vi "5-Axis (Manual).vi"() -> ()   [LabVIEW 2014]
uses:
  EMC API/EMC_Typedef_Motor_Parameters.ctl
  Typedef/Typedef_Motor_Action.ctl
  Functional_Global/Typedef_FPGA_Interface_Action.ctl
  <vilib>/Motion/Express/_s/nimc.ex.clearFaults.clearFaults.axis.vi
  <vilib>/Motion/Express/_s/nimc.ex.power.power.axis.vi
  <vilib>/Motion/Express/_s/nimc.ex.resetPosition.resetPosition.axis.vi
  <vilib>/Utility/error.llb/Error Cluster From Error Code.vi
  <vilib>/rvi/errors/niLvFpgaAdjustHostInterfaceError.vi
  <vilib>/Motion/Express/_s/nimc.ex.read.readTrajectoryData.axis.vi
  <vilib>/Motion/Express/_s/nimc.ex.read.readMotionIO.axis.vi
  <vilib>/Motion/Express/_s/nimc.ex.findReferenceMove.startReferenceMove.axis.modeReverseLimit.vi
  <vilib>/Motion/Express/_s/nimc.ex.findReferenceMove.startReferenceMove.axis.modeHome.vi
  <vilib>/Motion/Express/_s/nimc.ex.findReferenceMove.startReferenceMove.axis.modeForwardLimit.vi
  <vilib>/Motion/BlockNode/FB.NIMotion.xnode
  <vilib>/rvi/interface/nirviReadWriteControl/nirviReadWriteControl.xnode
  NiFpgaLv.dll
  <vilib>/rvi/interface/Simulation/niFpgaSimulationCallBeginRW.vi
panel:
  out "Rev Limits":bool[](array[boolean])
  out "Fwd Limits":bool[](array[boolean])
  out "Home Limits":bool[](array[boolean])
  in  "Mod3/DIO28":bool
  in  "Mod3/DIO29":bool
  in  "Mod3/DIO30":bool
  in  "Mod3/DIO31":bool
  in  "resource":refnum<k21>="Axis 1"
  out "home active":bool
  out "rev. limit active":bool
  out "fwd. limit active":bool
  out "XY Graph":cluster{"X Array":dbl[], "Y Array":dbl[]}(graph)
  in  "interval":dbl=0.01 format="%#_13g"
  in  "Gear in/out":enum16{"Gear in", "Gear out"}(ring)
  in  "denominator":i32=1
  in  "numerator":i32=1
  in  "Master Axis":T1(ring)
  out "Array":dbl[](array[knob]) scale=0.0..1000.0
  in  "Clear Errors":bool
  in  "Command":T2
  in  "Motion Parameters":T3={"position"=1000.0, "velocity"=1000.0, "acceleration"=10000.0, "deceleration"=10000.0, "accel. jerk"=10000.0, "decel. jerk"=10000.0}
  in  "Axis Index":T1(ring)
  out "error":errorcluster
  out "Numeric":i32
  in  "Stop all motors":bool
  in  "Execute Command":bool
  in  "stop":bool
  out "Axis Velocities":T4(graph)
  out "Axis Positions":T4(graph)
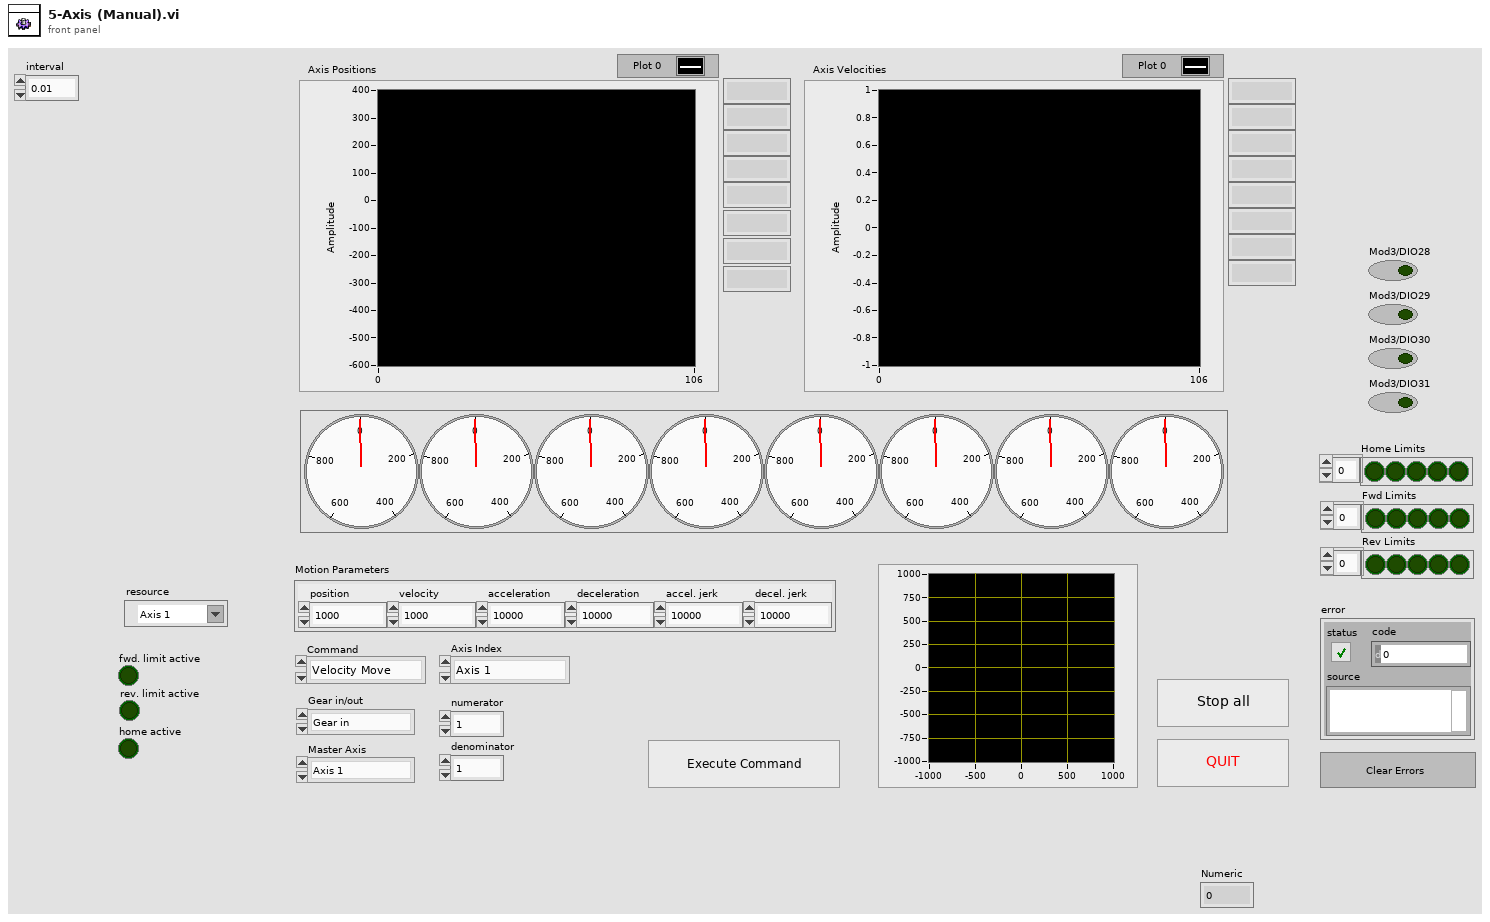
[diagram p1: front panel]
types:
  T1 = enum16{"Axis 1", "Axis 2", "Axis 3", "Axis 4", "Axis 5", "Axis 6", "Axis 7", "Axis 8"}
  T2 = typedef "Typedef_Motor_Action.ctl" = enum16{"Velocity Move", "REL Pos Move", "ABS Pos Move", "Stop", "Reset Position", "Coordinate_move", "Contour_move", "Gearing", "Find Fwd Limit", "Find Rev Limit", "Find Home"}
  T3 = typedef "EMC_Typedef_Motor_Parameters.ctl" = cluster{"position":dbl, "velocity":dbl, "acceleration":dbl, "deceleration":dbl, "accel. jerk":dbl, "decel. jerk":dbl}
  T4 = cluster{"[0]":dbl, "[1]":dbl, "[2]":dbl, "[3]":dbl, "[4]":dbl, "[5]":dbl, "[6]":dbl, "[7]":dbl}
  T5 = typedef "Typedef_FPGA_Interface_Action.ctl" = enum16{"Initialize FPGA", "Get FPGA Reference", "Close FPGA"}
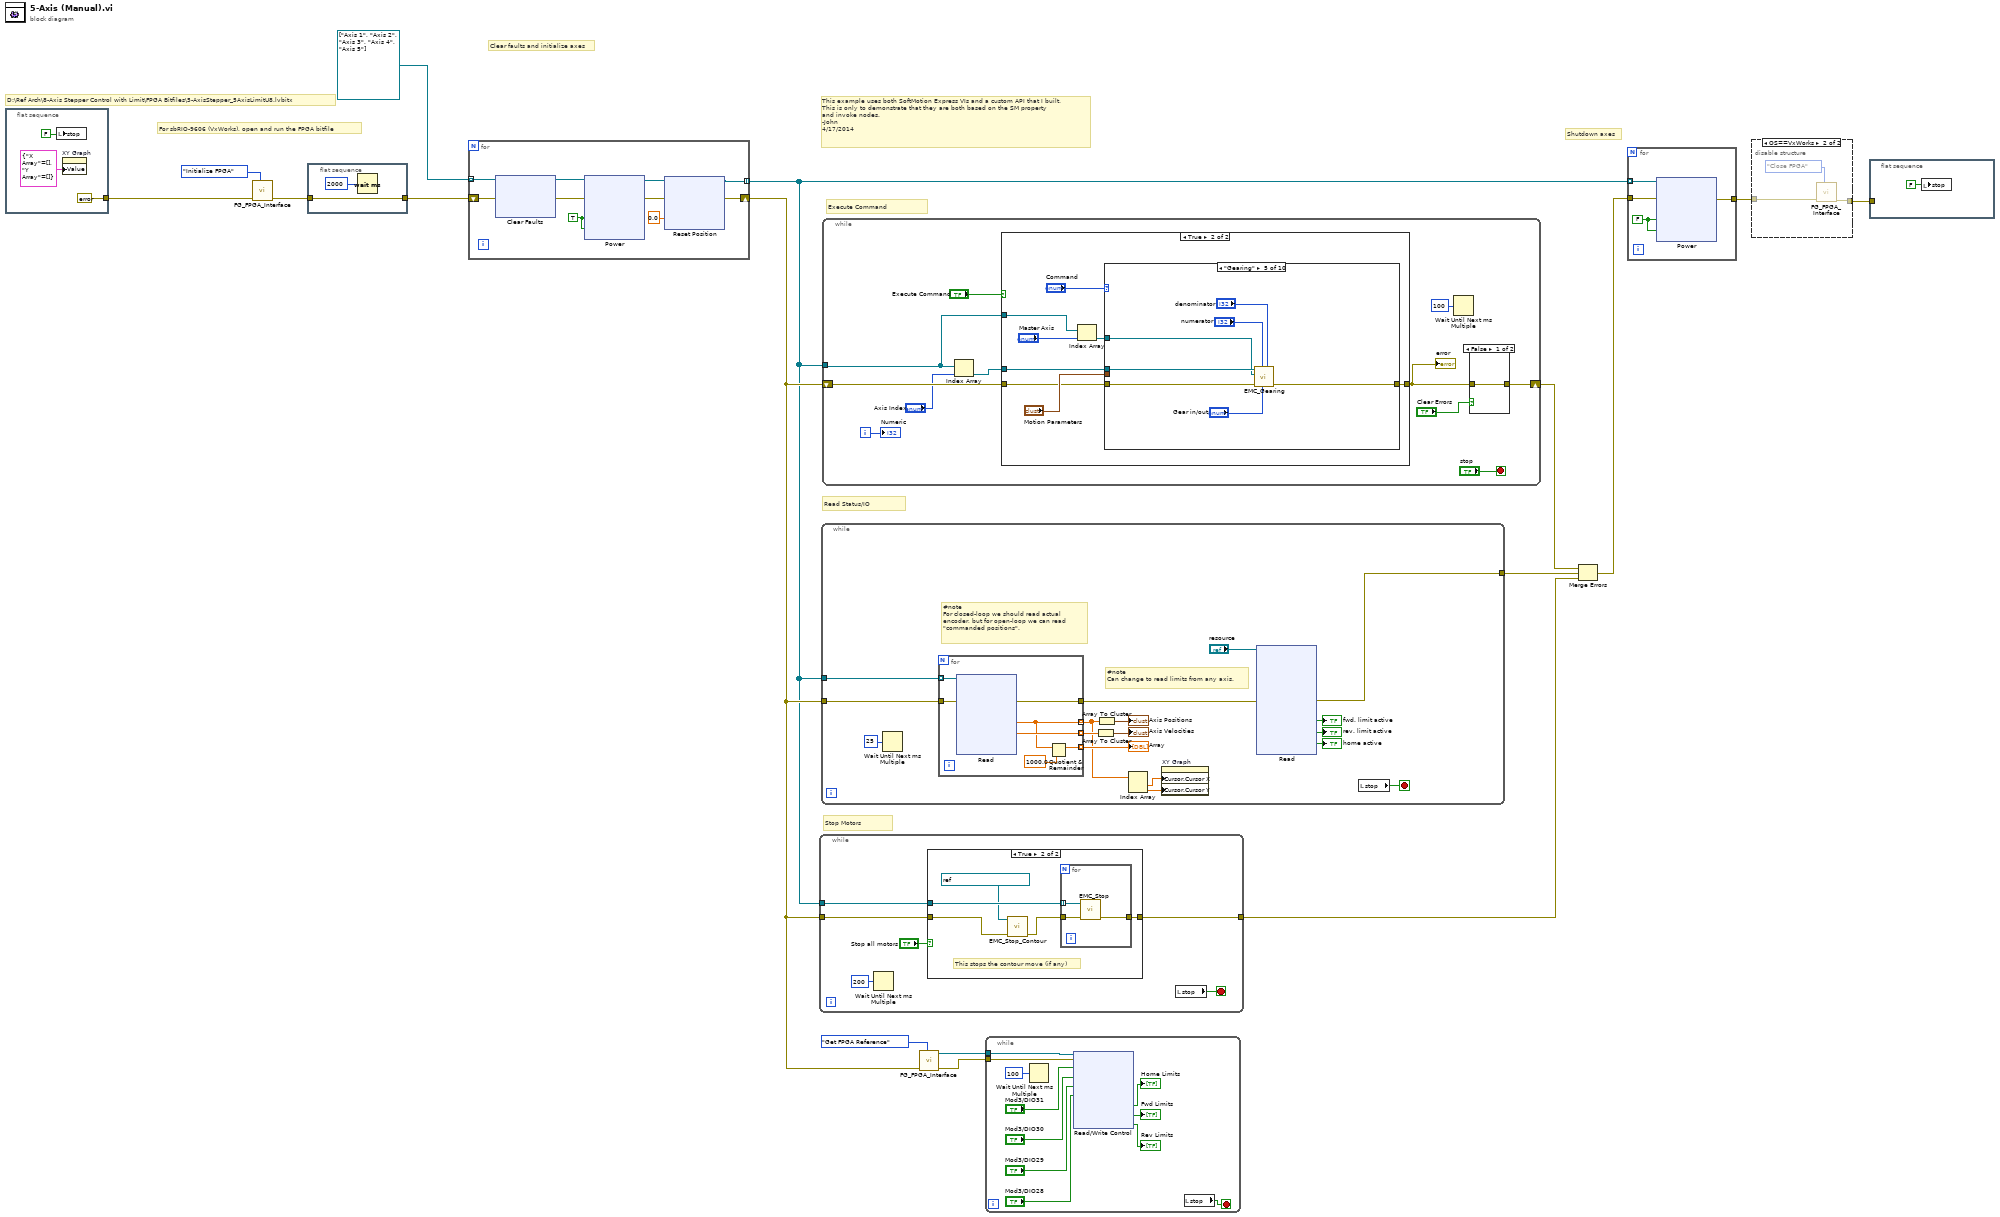
[diagram p0: block diagram]
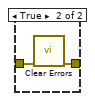
[diagram p4: hidden frame]
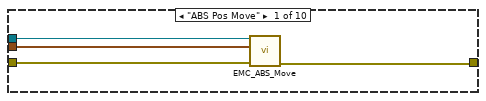
[diagram p6: hidden frame]
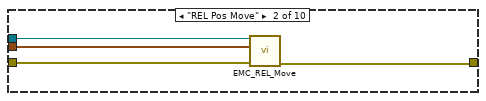
[diagram p7: hidden frame]
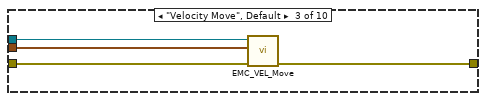
[diagram p8: hidden frame]
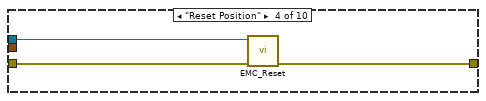
[diagram p9: hidden frame]
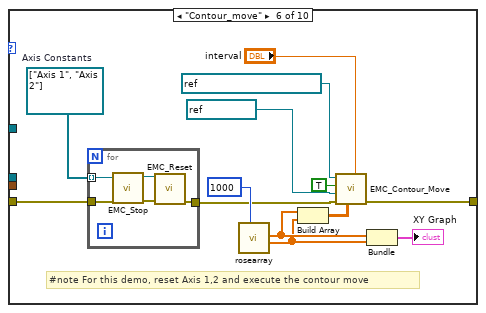
[diagram p10: hidden frame]
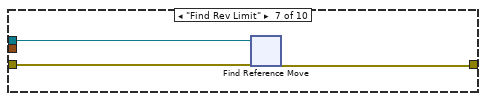
[diagram p11: hidden frame]
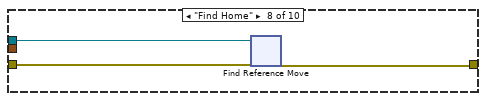
[diagram p12: hidden frame]
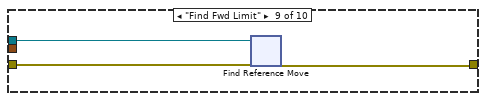
[diagram p13: hidden frame]
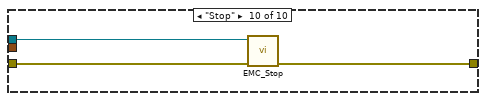
[diagram p14: hidden frame]
diagram:
  # "For sbRIO-9606 (VxWorks), open and run the FPGA bitfile"
  # "D:\\Ref Arch\\8-Axis Stepper Control with Limit\\FPGA Bitfiles\\5-AxisStepper_5AxisLimitU8.lvbitx"
  # "Clear faults and initialize axes"
  # "This example uses both SoftMotion Express VIs and a custom API that I built.\nThis is only to demonstrate that they are both based on the SM property\nand invoke nodes. \n-John\n4/17/2014"
  # "Shutdown axes"
  # "Execute Command"
  # "Read Status/IO"
  # "Stop Motors"
  n1 = flat-sequence {
    tunnel: [errorcluster {"status"=FALSE, "code"=0, "source"=""} ("error in (no error)")] -> w13
    frame #0 {
      n2 = local write "stop"(FALSE ("stop")) -> ()
      n3 = property on="XY Graph" class="XYGraph (strict)"("Value"=cluster{"X Array":dbl[], "Y Array":dbl[]} {"X Array"=[], "Y Array"=[]} ("XY Graph")) -> ()  [unwired: 2 in, 2 out]
    }
  }
  n4 = call "FG_FPGA_Interface.vi"("Action"=Typedef_FPGA_Interface_Action."Initialize FPGA", "error in"=w13) -> ("error out"=w8:errorcluster)  [unwired: 8 in, 1 out]
  n5 = flat-sequence {
    tunnel: w8 -> [w20]
    tunnel: [w20] -> w3
    frame #0 {
      n6 = Wait (ms)(milliseconds to wait=u32 2000) -> ()  [unwired: 1 out]
    }
  }
  n7 = for {
    tunnel: refnum<k21>[] ["Axis 1", "Axis 2", "Axis 3", "Axis 4", "Axis 5"] -> [w22] mode=indexing
    shift-right: [w31] -> w6
    shift-left: w3 -> [w25]
    tunnel: [w26] -> w1 mode=indexing
    w30 = TRUE ("enable axis")
    n8 = xnode ("Clear Faults")("resource"=w22, "error in"=w25) -> ("resource out"=w23:refnum<k21>, "error out"=w24:errorcluster)
    n9 = xnode ("Power")("enable axis"=w30, "enable drive"=w30, "resource"=w23, "error in"=w24) -> ("resource out"=w29:refnum<k21>, "error out"=w28:errorcluster)
    n10 = xnode ("Reset Position")("position"=0.0, "resource"=w29, "error in"=w28) -> ("resource out"=w26:refnum<k21>, "error out"=w31:errorcluster)
  }
  n11 = while {
    tunnel: w6 -> [w55]
    tunnel: w1 -> [w53]
    tunnel: [w51] -> w16
    stop <- w56 stop-if-true
    n12 = Wait Until Next ms Multiple(millisecond multiple=u32 200) -> ()  [unwired: 1 out]
    n13 = case shown="True" "Stop all motors" {
      tunnel: w55 -> [w57 w60]
      tunnel: [w57 w62] -> w51
      tunnel: w53 -> [_ w61]
      frame False {
      }
      frame True {
        # "This stops the contour move (if any)"
        n14 = call "EMC_Stop_Contour.vi"("error in (no error)"=w60, "coordinate"=refnum<k21> "Coordinate Space 1") -> ("error out"=w58:errorcluster)  [unwired: 9 in]
        n15 = for {
          tunnel: w58 -> [w65]
          tunnel: w61 -> [w63] mode=indexing
          tunnel: [w64] -> w62
          n16 = call "EMC_Stop.vi"("error in (no error)"=w65, "axis"=w63) -> ("error out"=w64:errorcluster)  [unwired: 8 in, 1 out]
        }
      }
    }
    n17 = local read "stop"() -> (w56:bool)
  }
  n18 = while {
    tunnel: w6 -> [w78]
    tunnel: w1 -> [w77]
    tunnel: [w66] -> w15
    stop <- w82 stop-if-true
    # "#note \nCan change to read limits from any axis."
    # "#note \nFor closed-loop we should read actual \nencoder, but for open-loop we can read\n\"commanded positions\"."
    n19 = Wait Until Next ms Multiple(millisecond multiple=u32 25) -> ()  [unwired: 1 out]
    n20 = for {
      tunnel: [w117] -> w68
      tunnel: [w112] -> w75 mode=indexing
      tunnel: [w116] -> w81 mode=indexing
      tunnel: w78 -> [w115]
      tunnel: w77 -> [w114] mode=indexing
      tunnel: [w111] -> w76 mode=indexing
      n21 = xnode ("Read")("resource"=w114, "error in"=w115) -> ("commanded position"=w112:dbl, "commanded vel."=w116:dbl, "error out"=w117:errorcluster)  [unwired: 2 out]
      n22 = Quotient & Remainder(x=w112, y=1000.0) -> (x-y*floor(x/y)=w111:dbl)  [unwired: 1 out]
    }
    "Array" <- w76
    n23 = Array To Cluster(array=w81) -> (cluster=→"Axis Velocities":T4)
    n24 = Array To Cluster(array=w75) -> (cluster=→"Axis Positions":T4)
    n25 = Index Array(array=w75) -> (element #1=w74:dbl, element #2=w73:dbl)  [unwired: 2 in]
    n26 = property on="XY Graph" class="XYGraph (strict)"("Cursor.Cursor X"=w74, "Cursor.Cursor Y"=w73) -> ()  [unwired: 2 in, 2 out]
    n27 = xnode ("Read")("resource"="resource", "error in"=w68) -> ("fwd. limit active"=→"fwd. limit active":bool, "rev. limit active"=→"rev. limit active":bool, "home active"=→"home active":bool, "error out"=w66:errorcluster)  [unwired: 6 out]
    n28 = local read "stop"() -> (w82:bool)
  }
  n29 = while {
    tunnel: w1 -> [w125]
    shift-right: [w126] -> w12
    shift-left: w6 -> [w130]
    i -> [w135]
    stop <- "stop" stop-if-true
    n30 = Index Array(array=w125, index="Axis Index") -> (element=w131:refnum<k21>)
    n31 = case shown="True" "Execute Command" {
      tunnel: w130 -> [w139 w146]
      tunnel: w131 -> [_ w145]
      tunnel: [w139 w144] -> w127
      tunnel: w125 -> [_ w141]
      frame False {
      }
      frame True {
        n32 = Index Array(array=w141, index="Master Axis") -> (element=w140:refnum<k21>)
        n33 = case shown="\"Gearing\"" "Command" {
          tunnel: "Motion Parameters" -> [w148 w152 w159 _ _ _ _ _ _ _]
          tunnel: w146 -> [w151 w155 w158 w162 w169 w172 w189 w208 w229 w249]
          tunnel: w145 -> [w149 w153 w157 w161 w168 _ w188 w207 w228 w247]
          tunnel: [w150 w154 w156 w160 w167 w182 w190 w209 w230 w248] -> w144
          tunnel: w140 -> [_ _ _ _ w163 _ _ _ _ _]
          frame "ABS Pos Move" {
            n34 = call "EMC_ABS_Move.vi"("error in (no error)"=w151, "Motion Parameters"=w148, "axis"=w149) -> ("error out"=w150:errorcluster)  [unwired: 8 in]
          }
          frame "REL Pos Move" {
            n35 = call "EMC_REL_Move.vi"("error in (no error)"=w155, "Motion Parameters"=w152, "axis"=w153) -> ("error out"=w154:errorcluster)  [unwired: 8 in]
          }
          frame "Velocity Move", Default {
            n36 = call "EMC_VEL_Move.vi"("error in (no error)"=w158, "Motion Parameters"=w159, "axis"=w157) -> ("error out"=w156:errorcluster)  [unwired: 8 in]
          }
          frame "Reset Position" {
            n37 = call "EMC_Reset.vi"("error in (no error)"=w162, "axis"=w161) -> ("error out"=w160:errorcluster)  [unwired: 9 in]
          }
          frame "Gearing" {
            n38 = call "EMC_Gearing.vi"("denominator"="denominator", "Gear in/out"="Gear in/out", "numerator"="numerator", "error in (no error)"=w169, "master axis"=w163, "axis"=w168) -> ("error out"=w167:errorcluster)  [unwired: 5 in]
          }
          frame "Contour_move" {
            w170 = refnum<k21>[] ["Axis 1", "Axis 2"]  # Axis Constants
            # "#note For this demo, reset Axis 1,2 and execute the contour move"
            n39 = for {
              tunnel: w172 -> [w186]
              tunnel: [w187] -> w171
              tunnel: w170 -> [w184] mode=indexing
              n40 = call "EMC_Stop.vi"("error in (no error)"=w186, "axis"=w184) -> ("error out"=w185:errorcluster, "axis out"=w183:refnum<k21>)  [unwired: 8 in]
              n41 = call "EMC_Reset.vi"("error in (no error)"=w185, "axis"=w183) -> ("error out"=w187:errorcluster)  [unwired: 9 in]
            }
            n42 = call "rosearray.vi"("Iterations"=u32 1000) -> ("Y Array"=w174:dbl[], "X Array"=w175:dbl[])  [unwired: 5 in, 1 out]
            n43 = Build Array(w175, w174) -> (w178:dbl[][])
            n44 = call "EMC_Contour_Move.vi"("interval"="interval", "points[][]"=w178, "error in (no error)"=w171, "table"=refnum<k21> "Table 1" ("resource"), "overwrite"=TRUE, "coordinate"=refnum<k21> "Coordinate Space 1" ("resource")) -> ("error out"=w182:errorcluster)  [unwired: 5 in]
            n45 = Bundle("X Array"=w175, "Y Array"=w174) -> (→"XY Graph":cluster{"X Array":dbl[], "Y Array":dbl[]})  [unwired: 1 in]
          }
          frame "Find Rev Limit" {
            n46 = xnode "Find Reference Move"("resource"=w188, "error in"=w189) -> ("error out"=w190:errorcluster)  [unwired: 9 in, 2 out]
          }
          frame "Find Home" {
            n47 = xnode "Find Reference Move"("resource"=w207, "error in"=w208) -> ("error out"=w209:errorcluster)  [unwired: 11 in, 2 out]
          }
          frame "Find Fwd Limit" {
            n48 = xnode "Find Reference Move"("resource"=w228, "error in"=w229) -> ("error out"=w230:errorcluster)  [unwired: 9 in, 2 out]
          }
          frame "Stop" {
            n49 = call "EMC_Stop.vi"("error in (no error)"=w249, "axis"=w247) -> ("error out"=w248:errorcluster)  [unwired: 8 in, 1 out]
          }
        }
      }
    }
    "error" <- w127
    n50 = Wait Until Next ms Multiple(millisecond multiple=u32 100) -> ()  [unwired: 1 out]
    n51 = case shown="False" "Clear Errors" {
      tunnel: w127 -> [w136 w138]
      tunnel: [w136 w137] -> w126
      frame False {
      }
      frame True {
        n52 = call <vilib>:"Clear Errors.vi"("error in (no error)"=w138) -> ("error out"=w137:errorcluster)  [unwired: 5 in, 1 out]
      }
    }
    "Numeric" <- w135
  }
  n53 = call "FG_FPGA_Interface.vi"("Action"=Typedef_FPGA_Interface_Action."Get FPGA Reference", "error in"=w6) -> ("error out"=w5:errorcluster, "FPGA VI Reference Out"=w4:refnum<k20>)  [unwired: 8 in]
  n54 = while {
    tunnel: w5 -> [w259]
    tunnel: w4 -> [w260]
    stop <- w250 stop-if-true
    n55 = Wait Until Next ms Multiple(millisecond multiple=u32 100) -> ()  [unwired: 1 out]
    n56 = xnode "Read/Write Control"("FPGA VI Reference In"=w260, "error in"=w259, "Mod3/DIO31"="Mod3/DIO31", "Mod3/DIO30"="Mod3/DIO30", "Mod3/DIO29"="Mod3/DIO29", "Mod3/DIO28"="Mod3/DIO28") -> ("Home Limits"=→"Home Limits":bool[], "Fwd Limits"=→"Fwd Limits":bool[], "Rev Limits"=→"Rev Limits":bool[])  [unwired: 2 out]
    n57 = local read "stop"() -> (w250:bool)
  }
  n58 = Merge Errors(w12, w15, w16) -> (w11:errorcluster)
  n59 = for {
    tunnel: w1 -> [w264] mode=indexing
    tunnel: [w262] -> w10
    tunnel: w11 -> [w261]
    w263 = FALSE ("enable axis")
    n60 = xnode ("Power")("enable axis"=w263, "enable drive"=w263, "resource"=w264, "error in"=w261) -> ("error out"=w262:errorcluster)  [unwired: 1 out]
  }
  n61 = disable-structure shown="OS==VxWorks" {
    disable-tunnel: w10 -> [w275 w277]
    disable-tunnel: [w275 w276] -> w14
    frame condition #0 (active) {
    }
    frame condition #1 {
      n62 = call "FG_FPGA_Interface.vi"("Action"=Typedef_FPGA_Interface_Action."Close FPGA", "error in"=w277) -> ("error out"=w276:errorcluster)  [unwired: 8 in, 1 out]
    }
  }
  n63 = flat-sequence {
    tunnel: w14 -> [_]
    frame #0 {
      n64 = local write "stop"(FALSE ("stop")) -> ()
    }
  }
